vi "UTIL Probe.vi"(8 "error in (no error)":errorcluster, 11 "niDTS Comm Telnet in":refnum<class "niDTS Comm Telnet.lvclass">) -> (0 "error out":errorcluster, 3 "niDTS Comm Telnet out":refnum<class "niDTS Comm Telnet.lvclass">)   [LabVIEW 2015, in "niDTS CommLib.lvlib" / "niDTS Comm Telnet.lvclass"]
uses:
  niDTS Comm Telnet.lvclass
  Includes/niDTS Comm INC Telnet Port Parameters.ctl
  Utility/telnet/telnet.llb/Telnet Session.ctl
  niDTS Comm Telnet.lvclass/niDTS Comm Telnet.ctl
  niDTS CommLib.lvlib
panel:
  out "IP Address":string="192.168.1.200"
  out "Telnet Reference":T1
  out "Port Parameters":T2={"Bytes to Read"=1000, "Line Separator"="\n", "Port Timeout (ms)"=5000, "Read Mode"=enum."normal", "Write Mode"=enum."normal", "Remote Port"=23}
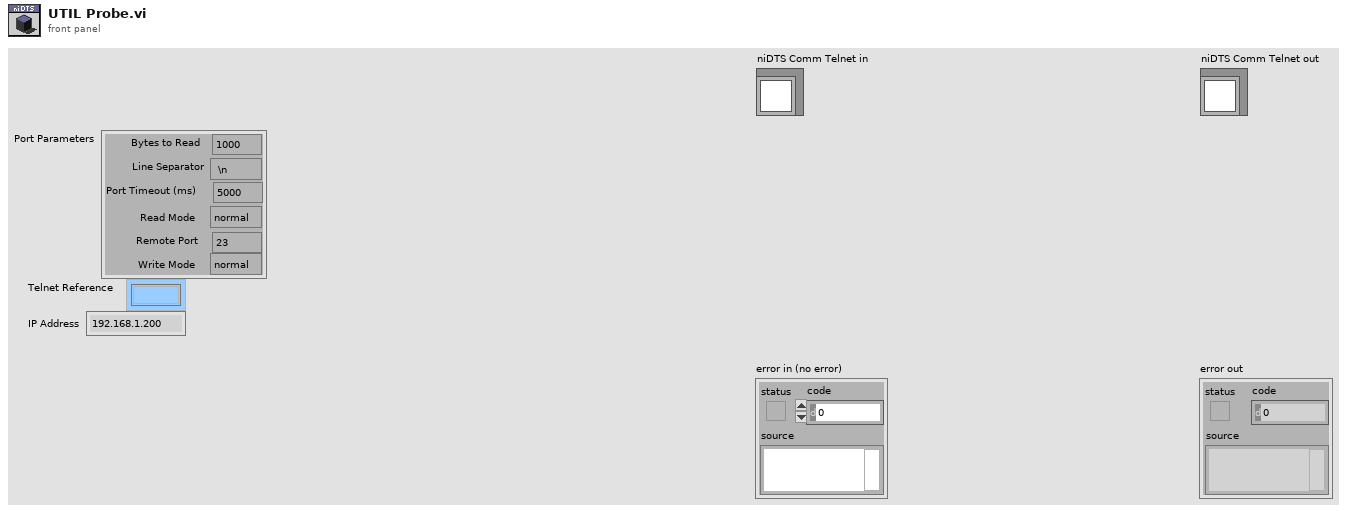
[diagram p1: front panel]
types:
  T1 = typedef "Telnet Session.ctl" = refnum<k1>
  T2 = typedef "niDTS CommLib.lvlib/niDTS Comm INC Telnet Port Parameters.ctl" = cluster{"Bytes to Read":i32, "Line Separator":string, "Port Timeout (ms)":i32, "Read Mode":enum16{"normal", "line", "buffered"}, "Write Mode":enum16{"normal", "line", "buffered"}, "Remote Port":u16}
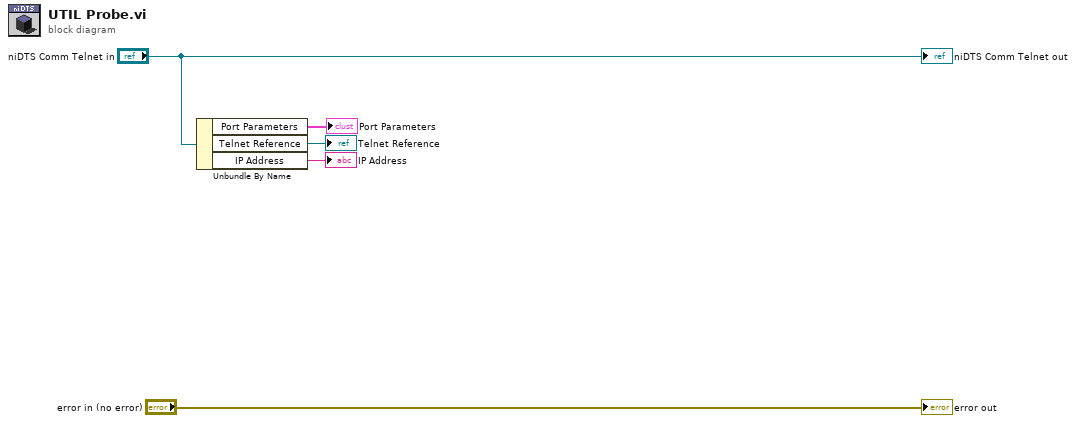
[diagram p0: block diagram]
diagram:
  n1 = Unbundle By Name("niDTS Comm Telnet in") -> ("Port Parameters"=→"Port Parameters":T2, "Telnet Reference"=→"Telnet Reference":T1, "IP Address"=→"IP Address":string)
  "error out" <- "error in (no error)"
  "niDTS Comm Telnet out" <- "niDTS Comm Telnet in"
